vi "Property required.vi"(8 "error in (no error)":errorcluster, 9 "Name":string, 10 "Required?":bool, 11 "JSON Schema in":string) -> (0 "error out":errorcluster, 3 "JSON Schema out":string)   [LabVIEW 2023, in "JSON Schema Generator.lvlib"]
uses:
  JSON Schema Generator.lvlib
  d81358e3-cc5e-48f6-8576-1aee33a06cd4.vi
  <vilib>/JDP Science/JSONtext/Next JSON Value.vi
  <vilib>/JDP Science/JSONtext/String Subset.vi
  <vilib>/JDP Science/JSONtext/Parsing/Advance past next JSON Value (inlined COPY).vi
  <vilib>/JDP Science/JSONtext/Parsing/Advance past whitespace.vi
  <vilib>/JDP Science/JSONtext/Parsing/Advance past String.vi
  <vilib>/JDP Science/JSONtext/Parsing/Advance past Number.vi
  <vilib>/JDP Science/JSONtext/Parsing/Advance past Line Ending.vi
  <vilib>/JDP Science/JSONtext/Variant to JSON Text.vi
  <vilib>/JDP Science/JSONtext/Parsing/Parse Full Path or Item Name.vi
  <vilib>/JDP Science/JSONtext/Parsing/Advance past Array.vi
  <vilib>/JDP Science/JSONtext/Parsing/Advance past Object.vi
  <vilib>/JDP Science/JSONtext/support/Error Cluster From Code.vi
  <vilib>/JDP Science/JSONtext/Offset/Find Item Locations by Path.vi
  <vilib>/JDP Science/JSONtext/support/Format JSON Array Text.vi
  <vilib>/JDP Science/JSONtext/LVClass Serializer/JSONtext LVClass Serializer.lvclass
  <vilib>/JDP Science/JSONtext/JSONtext.lvlib
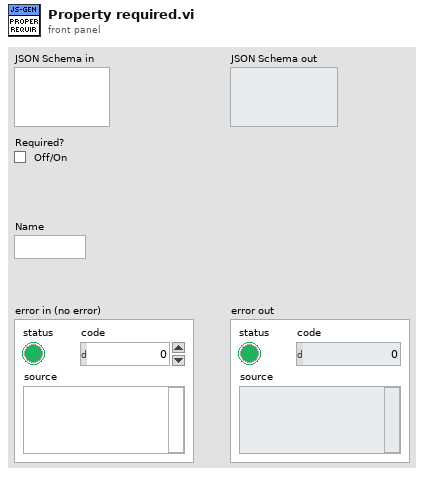
[diagram p1: front panel]
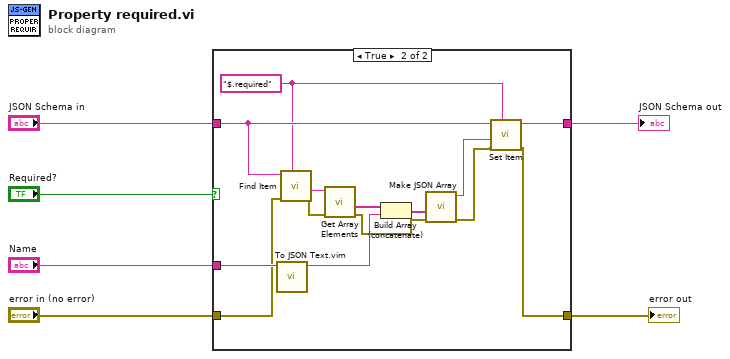
[diagram p0: block diagram]
diagram:
  n1 = case shown="True" "Required?" {
    tunnel: "JSON Schema in" -> [w8 w20]
    tunnel: [w8 w22] -> w3
    tunnel: "Name" -> [_ w15]
    tunnel: [w7 w21] -> w6
    tunnel: "error in (no error)" -> [w7 w9]
    frame False {
    }
    frame True {
      w19 = "$.required" ("$Path or Item Name")
      n2 = call "To JSON Text.vim"("Anything"=w15) -> ("<JSON>"=w10:string)  [unwired: 9 in, 1 out]
      n3 = call <vilib>:"Find Item.vi"("$Path or Item Name"=w19, "error in (no error)"=w9, "JSON"=w20) -> ("error out"=w13:errorcluster, "<JSON>"=w18:string)  [unwired: 5 in, 2 out]
      n4 = call <vilib>:"Get Array Elements.vi"("error in (no error)"=w13, "JSON"=w18) -> ("error out"=w12:errorcluster, "<JSON>"=w17:string[])  [unwired: 7 in, 1 out]
      n5 = Build Array (concatenate)(w17, w10) -> (w16:string[])
      n6 = call <vilib>:"Make JSON Array.vi"("error in (no error)"=w12, "JSON Elements"=w16) -> ("error out"=w11:errorcluster, "<JSON>"=w14:string)  [unwired: 8 in]
      n7 = call <vilib>:"Set Item.vi"("$Path or Item Name"=w19, "error in (no error)"=w11, "JSON to Insert"=w14, "JSON"=w20) -> ("error out"=w21:errorcluster, "<JSON>"=w22:string)  [unwired: 4 in, 1 out]
    }
  }
  "error out" <- w6
  "JSON Schema out" <- w3
